vi "Run Command.vi"(2 "Line Index In":i32, 3 "Script":string) -> (0 "Line Index Out":i32, 1 "Done":bool)   [LabVIEW 2018]
doc: "Looks at a line and runs the appropriate command. Add new commands to this vi."
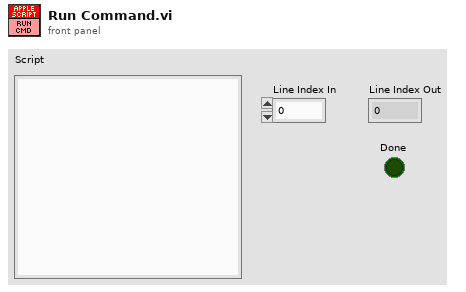
[diagram p1: front panel]
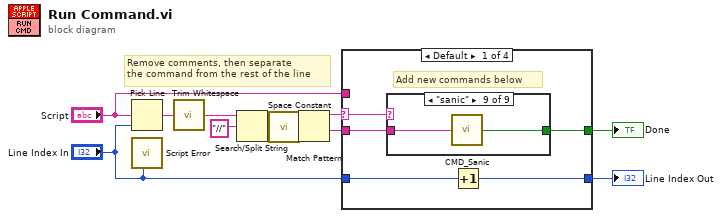
[diagram p0: block diagram]
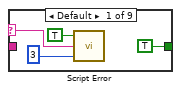
[diagram p2: hidden frame]
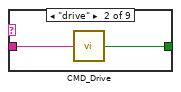
[diagram p3: hidden frame]
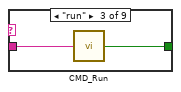
[diagram p4: hidden frame]
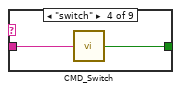
[diagram p5: hidden frame]
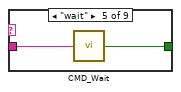
[diagram p6: hidden frame]
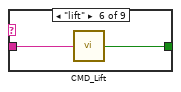
[diagram p7: hidden frame]
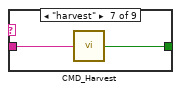
[diagram p8: hidden frame]
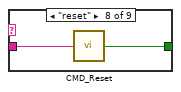
[diagram p9: hidden frame]
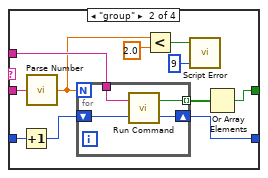
[diagram p10: hidden frame]
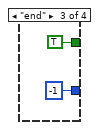
[diagram p11: hidden frame]
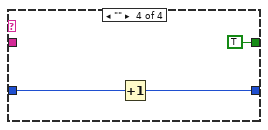
[diagram p12: hidden frame]
diagram:
  # "Remove comments, then separate\nthe command from the rest of the line"
  n1 = Pick Line(multi-line string="Script", line index="Line Index In") -> (output string=w6:string)  [unwired: 1 in]
  n2 = call "Script Error.vi"("Line Number"="Line Index In") -> ()  [unwired: 4 in, 1 out]
  n3 = call <vilib>:"Trim Whitespace.vi"("string"=w6) -> ("trimmed string"=w4:string)  [unwired: 1 in]
  n4 = Search/Split String(string=w4, search string/char (-)="//") -> (substring before match=w3:string)  [unwired: 1 in, 2 out]
  n5 = call <vilib>:"Space Constant.vi"() -> ("String"=w11:string)
  n6 = Match Pattern(string=w3, regular expression=w11) -> (before substring=w2:string, after substring=w1:string)  [unwired: 1 in, 2 out]
  n7 = case shown="Default" w2 {
    selector: w2 -> [w14 _ _ _]
    tunnel: "Script" -> [_ w47 _ _]
    tunnel: "Line Index In" -> [w16 w43 _ w55]
    tunnel: [w13 w45 TRUE ("Running") TRUE ("Running")] -> w9
    tunnel: [w15 w44 -1 ("Line Index Out") w54] -> w8
    tunnel: w1 -> [w12 w37 _ _]
    frame Default {
      # "Add new commands below"
      n8 = case shown="\"sanic\"" w14 {
        selector: w14 -> [w17 _ _ _ _ _ _ _ _]
        tunnel: [TRUE w22 w23 w26 w28 w30 w32 w34 w36] -> w13
        tunnel: w12 -> [_ w21 w24 w25 w27 w29 w31 w33 w35]
        frame Default {
          n9 = call "Script Error.vi"("Error?"=TRUE, "Error Details"=w17, "Error Code"=3) -> ()  [unwired: 2 in, 1 out]
        }
        frame "drive" {
          n10 = call "CMD_Drive.vi"("Line"=w21) -> ("Done"=w22:bool)
        }
        frame "run" {
          n11 = call "CMD_Run.vi"("Line"=w24) -> ("Done"=w23:bool)
        }
        frame "switch" {
          n12 = call "CMD_Switch.vi"("Line"=w25) -> ("Done"=w26:bool)
        }
        frame "wait" {
          n13 = call "CMD_Wait.vi"("Line"=w27) -> ("Done"=w28:bool)
        }
        frame "lift" {
          n14 = call "CMD_Lift.vi"("Line"=w29) -> ("Done"=w30:bool)
        }
        frame "harvest" {
          n15 = call "CMD_Harvest.vi"("Line"=w31) -> ("Done"=w32:bool)
        }
        frame "reset" {
          n16 = call "CMD_Reset.vi"("Line"=w33) -> ("Done"=w34:bool)
        }
        frame "sanic" {
          n17 = call "CMD_Sanic.vi"("Line"=w35) -> ("Done"=w36:bool)
        }
      }
      n18 = Increment(x=w16) -> (x+1=w15:i32)
    }
    frame "group" {
      n19 = Increment(x=w43) -> (x+1=w42:i32)
      n20 = call "Parse Number.vi"("String"=w37) -> ("Number"=w40:dbl)
      n21 = for {
        N: w40 -> [_]
        tunnel: w47 -> [w51]
        tunnel: [w50] -> w46 mode=indexing
        shift-right: [w49] -> w44
        shift-left: w42 -> [w48]
        n22 = call "Run Command.vi"("Line Index In"=w48, "Script"=w51) -> ("Line Index Out"=w49:i32, "Done"=w50:bool)
      }
      n23 = Less?(x=w40, y=2.0) -> (x < y?=w39:bool)
      n24 = call "Script Error.vi"("Error?"=w39, "Error Code"=9) -> ()  [unwired: 3 in, 1 out]
      n25 = Or Array Elements(Boolean array=w46) -> (logical OR=w45:bool)
    }
    frame "end" {
    }
    frame "" {
      n26 = Increment(x=w55) -> (x+1=w54:i32)
    }
  }
  "Line Index Out" <- w8
  "Done" <- w9
